vi "AlliGator Export Dataset to TIFF or HDF5.vi"(5 "Dialog?":bool, 6 "Gate Names (Gate)":string[](array[string]), 7 "Destination File Type":string, 8 "error in (no error)":errorcluster, 9 "Channel 2 Image Array":T2[](array[typedef]), 10 "Channel 1 Image Array":T2[](array[typedef]), 11 "Dataset Information":T1={"Single Point Data Path"=path "", "Dataset Timestamp (s)"=0.0, "Current Data"=""}) -> (0 "error out":errorcluster, 1 "Output String":string, 3 "File Path out":path)   [LabVIEW 2021, in "AlliGator Files.lvlib"]
doc: "Saves gate images and dataset information to either a HDF5 file or an image series.\n\n<B>Destination File Type</B>: 'TIFF Series' (Default) or 'HDF5'\n\nNote: TIFF Series does not support dual-gate datasets."
uses:
  AlliGator Files.lvlib
  <vilib>/vision/Image Controls.llb/IMAQ Image.ctl
  AlliGator Current Dataset Information.ctl
  AlliGator Saved TIFF Image Type.ctl
  AlliGator Saved Dataset Information.ctl
  Phasor/Phasor Fluorescence Lifetime Parameters v3.ctl
  Globals, Variables, Constants/AlliGator Variables List.ctl
  <vilib>/Utility/error.llb/Error Cluster From Error Code.vi
  Variant/Variant to Data/Variant to String.vi
  Variant/Variant to Data/Variant to I32.vi
  Globals, Variables, Constants/AlliGator Globals.vi
  <vilib>/ErrorRing/Error Ring.xnode
  GUI/GUI.lvlib
  HDF5/AlliGator HDF5.lvlib
  Strings/Strings.lvlib
  Globals, Variables, Constants/AlliGator Globals, Variables & Constants.lvlib
  Phasor/Phasor.lvlib
  Variant/Variant to Data/Variant to Data.lvlib
panel:
  # "see the AlliGator License on the block diagram (Ctrl+E or Window:Show Block Diagram)"
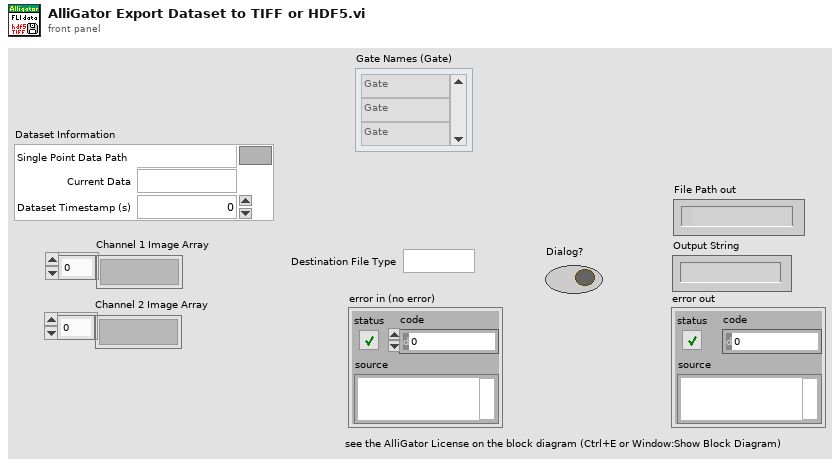
[diagram p1: front panel]
types:
  T1 = typedef "AlliGator Files.lvlib/AlliGator Current Dataset Information.ctl" = cluster{"Single Point Data Path":path, "Dataset Timestamp (s)":dbl, "Current Data":string}
  T2 = typedef "IMAQ Image.ctl" = refnum<image>
  T3 = typedef "Phasor.lvlib/Phasor Fluorescence Lifetime Parameters v3.ctl" = cluster{"# Pixel X":i32, "# Pixel Y":i32, "# Gates":i32, "# Datasets":i32, "Gate Image Exposure":dbl[unit], "Macrotime Gate Separation":dbl[unit], "Nanotime Gate Separation":dbl[unit], "Gate Width":dbl[unit], "Laser Period":dbl[unit], "SYNC Period":dbl[unit], "Gate Image Integration":dbl[unit]}
  T4 = cluster{"Gate Image File Name":string, "File Number Format":string, "Start Index":u32}
  T5 = typedef "AlliGator Files.lvlib/AlliGator Saved TIFF Image Type.ctl" = enum16{"Single Gate", "Sum of All Gates", "Phasor"}
  T6 = typedef "AlliGator Globals, Variables & Constants.lvlib/AlliGator Variables List.ctl" = enum16{"---- GUI ----", "GUI:Initialization Status", "GUI:State Indicators Refnum", "GUI:Original AlliGator Menu Items", "GUI:Current Action Loop State", "GUI:Script in progress", "GUI:Playback", "GUI:Loop Playback", "GUI:Search ROI Used", "GUI:Search ROI", "Decay Graph Max Legend Size", "Intensity Graph Max Legend Size", "Decay Statistics Graph Max Legend Size", "Phasor Graph Max Legend Size", "Phasor Ratio Graph Max Legend Size", "Lifetime Graph Max Legend Size", "---- Files ----", "Files:Export Dataset Frames as Individual Files", "Files:Show Batch Export Help Balloons", "Files:Frames in Dataset", "Files:ptu File Frame Start Indices", "Files:Current Frame in Dataset", "Files:Current Frame Timestamp", "Files:Dataset Loaded", "Files:Dataset Metadata", "Files:Dataset Channel", "Files:Dataset Data Description", "Files:Background Dataset Metadata", "Files:Background Dataset Channel", "Files:Background Dataset Data Description", "Files:Background File Subtraction", "Files:Background File Path", "Files:Background File Pile-up Correction", "Files:Background File Pixel Well Capacity", "Files:Background File Scaling Factor", "Files:Current Dataset Load Settings", "Files:Dataset Path", "Files:ICCD-specific Information", "Files:Macrotime Gate Separation", "------ Python Plugins ------", "Python Plugins:Information", "Python Plugins:Python Session", "Python Plugins:Valid Python Session?", "---- Source Image ----", "Source Image:ROIs", "Source Image:Current ROI", "Source Image:ROI Event Refnum", "X_Source Image:Display Range", "X_Source Image:Palette Information", "X_Source Image:Type of Displayed Image", "X_Time Gate Slider", "Source Image:Palette List", "Source Image:Scale", "Source Image:ROI Overlay Color", "Source Image:Overlay to Erase", "Source Image:Is Displayed Image Accumulated", "Source Image:White Light Image Modified", "Source Image:Mask Image Modified", "---- Image Profile Window ----", "Image Profile:Window Event Refnum", "Image Profile:IntensityType", "Image Profile:Intensity Average Type", "Image Profile:Intensity-weighted SDV", "Image Profile:Box Profile Type", "Image Profile:Window Open", "Image Profile:Plotted Fit Parameter", "------ Phasor Graph -------", "Phasor Graph:Show Line", "---- Phasor Plot ---", "Phasor Plot:Parameters Changed", "Phasor Plot:FLI Dataset Modified since last Calculation", "Phasor Harmonics Data", "Selected Phasor Harmonics", "Phasor Harmonic Manager Event Refnum", "Phasor Plot:ROIs", "Phasor Plot:Current ROI", "Phasor Plot:ROI Event Refnum", "Phasor Plot:Image Reference Points", "Phasor Plot:Computed", "Phasor Plot:Palette Information", "Phasor Plot:Palette List", "Phasor Plot:Phasor Ratio Palette Information", "Phasor Plot:Phasor Ratio Palette List", "Phasor Plot:Image Scale", "Phasor Plot:Image Overlay to Erase", "Phasor Plot:Image Elements to Update", "Phasor Plot:Current Calculation Parameters", "Phasor Plot:Current Calibration Options", "Phasor Plot:Reset Cumulated Phasor Plot", "Phasor Plot:Reference 1", "Phasor Plot:Lifetime Reference 1", "Phasor Plot:Reference 1 Frequency", "Phasor Plot:Reference 2", "Phasor Plot:Lifetime Reference 2", "Phasor Plot:Reference 2 Frequency", "---- Decay Analysis ----", "Number of Selected Decays to Fit", "LS Fit Results", "LAR Fit Results", "BS Fit Results", "Last Decay Max - Min", "Best Fit Parameters", "Best Fit Parameter Names", "Actual Size X", "Actual Size Y", "Binning X", "Binning Y", "Actual # Gates", "Dataset Number", "Gates to...", "Gates Skipped", "Gates to keep", "Gate Step", "Gate Separation", "Reversed Gates", "Pile-up Correction", "Pixel Well Capacity", "Background Subtracted", "Background Subtraction Method", "Background Definition Range", "Background File (deprecated)", "Number of Dataset Accumulated", "Array of Accumulated Dataset Paths", "Do Averaged Datasets", "Destination File Path", "Process Plot Target", "Use 1/D as Phasor Frequency", "---- Decay Fit Parameter Map -----", "Decay Fit Parameter Map:Palette Information", "Decay Fit Parameter Map:Palette List", "---- Parameter Map ----", "Parameter Map:Palette Information", "Parameter Map:Palette List", "------- Local Decay Window ---------", "Local Decay Graph Window:Event Refnum", "Local Decay Graph Window:Use normalized IRF for convolution", "----- Miscellaneous ----", "Misc:Skippable Dialog Windows Status"}
  T7 = typedef "AlliGator Files.lvlib/AlliGator Saved Dataset Information.ctl" = cluster{"Single Dataset Path":path, "Dataset ID in Series (1)":i32, "# Datasets in Series (1)":i32, "Dataset Timestamp (s)":dbl, "Additional Metadata":string, "DAQ Parameters":T3, "Dataset Data Description":string, "X Bin":i32, "Y Bin":i32}
  T8 = typedef "AlliGator Files.lvlib/AlliGator TIFF Series Options.ctl" = cluster{"Gate Image File Name":string, "File Number Format":string, "Start Index":u32, "Save Metadata File":bool, "Compress Image":bool}
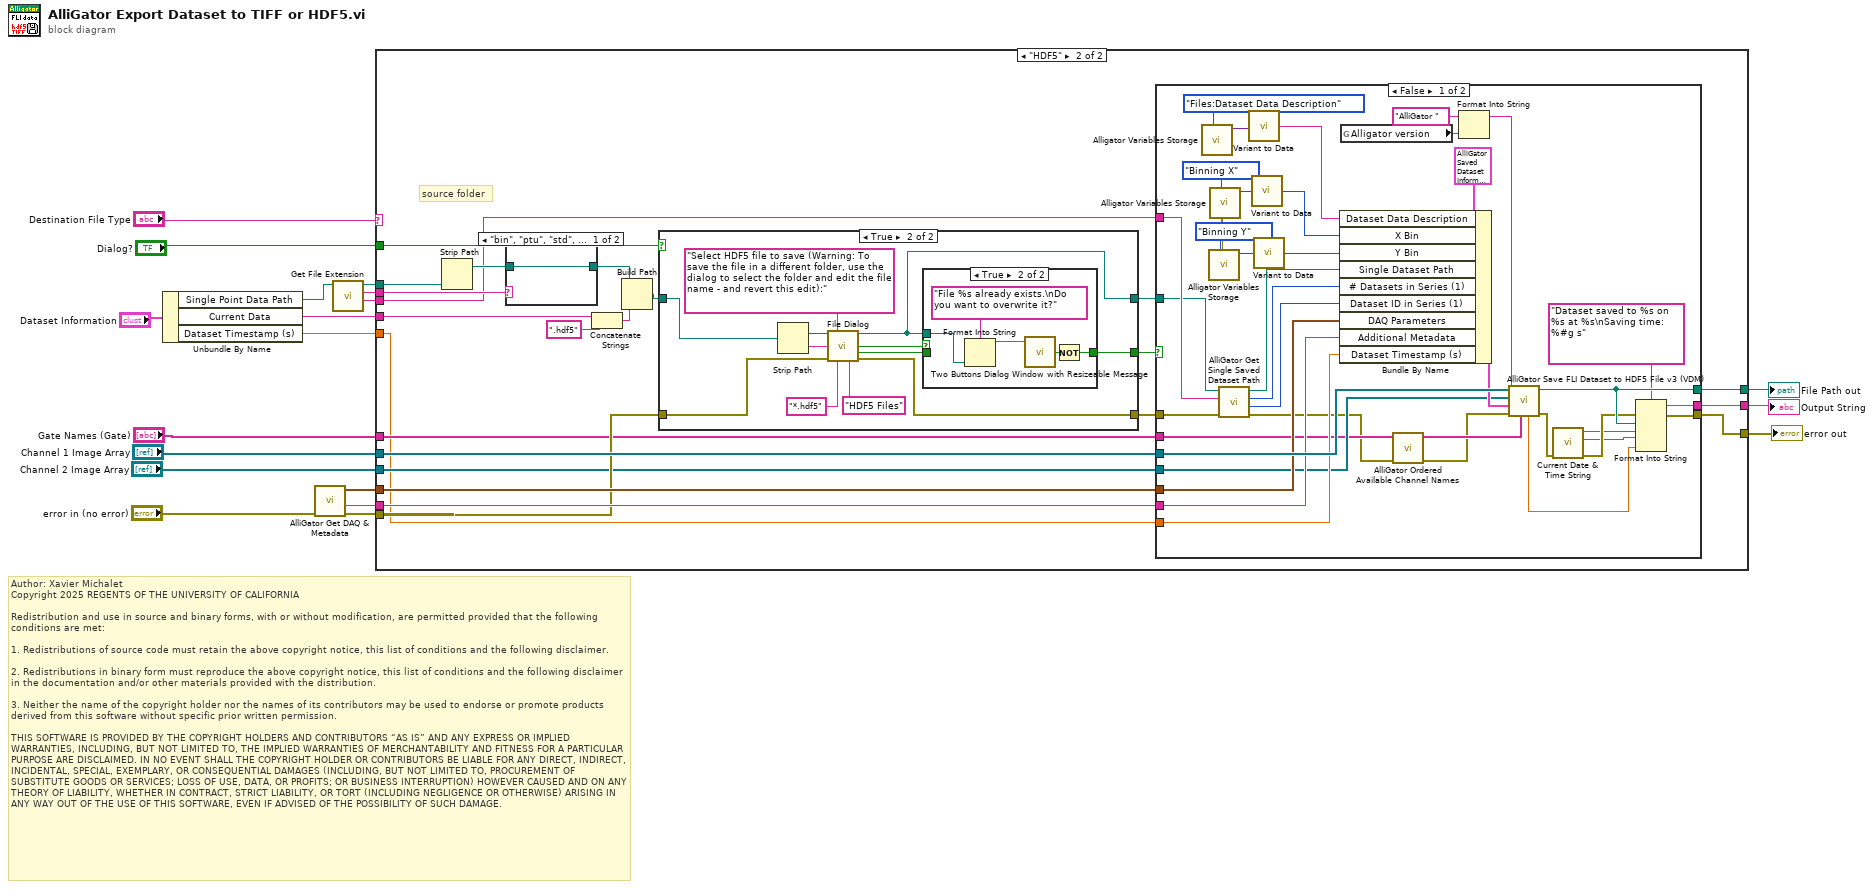
[diagram p0: block diagram]
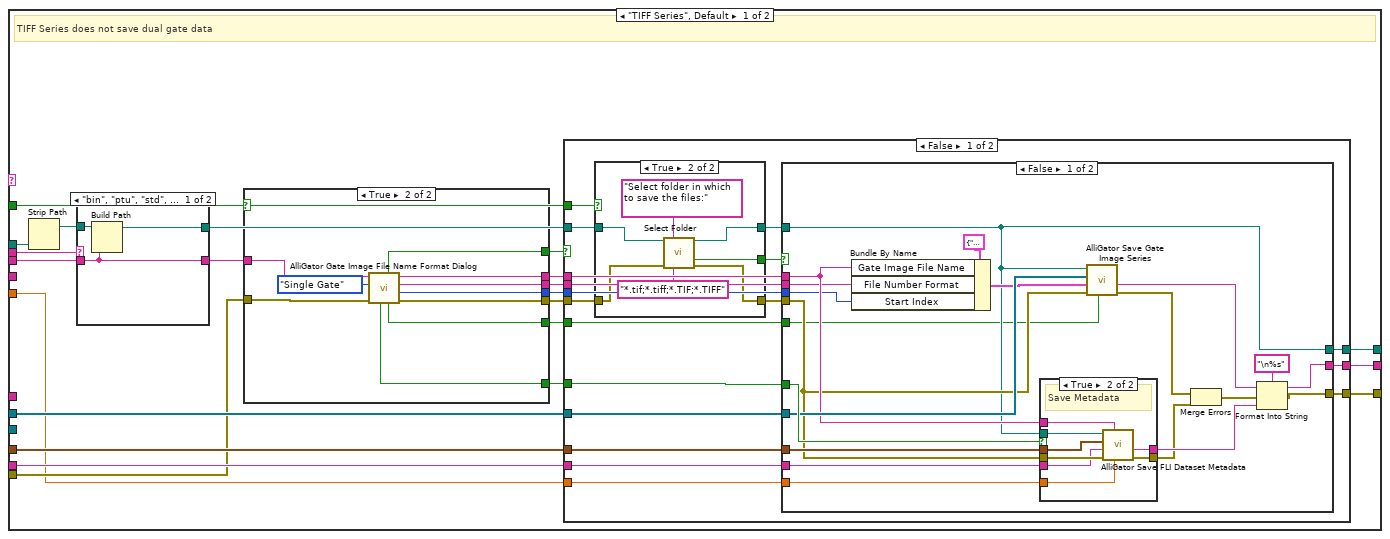
[diagram p2: hidden frame]
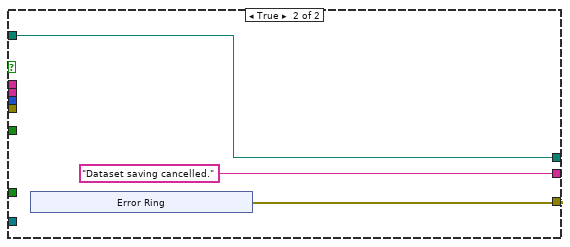
[diagram p4: hidden frame]
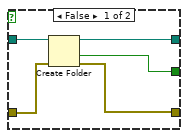
[diagram p5: hidden frame]
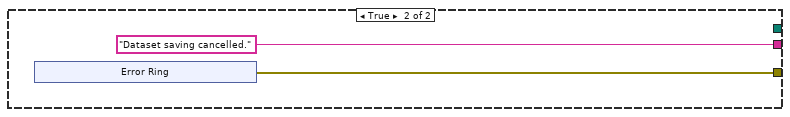
[diagram p6: hidden frame]
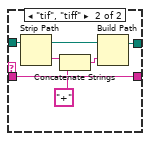
[diagram p7: hidden frame]
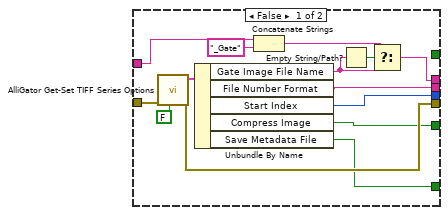
[diagram p8: hidden frame]
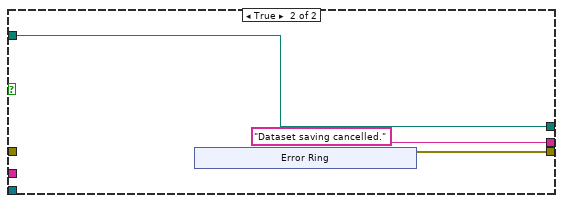
[diagram p9: hidden frame]
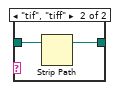
[diagram p12: hidden frame]
diagram:
  # "Author: Xavier Michalet\nCopyright 2025 REGENTS OF THE UNIVERSITY OF CALIFORNIA\n\nRedistribution and use in source and binary forms, with or without modification, are permitted provided that the following conditions are met:\n\n1. Redistributions of source code must retain the above copyright notice, this list of conditions and the following disclaimer.\n\n2. Redistributions in binary form must reproduce the above copyright notice, this list of conditions and the following disclaimer in the documentation and/or other materials provided with the distribution.\n\n3. Neither the name of the copyright holder nor the names of its contributors may be used to endorse or promote products derived from this software without specific prior written permission.\n\nTHIS SOFTWARE IS PROVIDED BY THE COPYRIGHT HOLDERS AND CONTRIBUTORS “AS IS” AND ANY EXPRESS OR IMPLIED WARRANTIES, INCLUDING, BUT NOT LIMITED TO, THE IMPLIED WARRANTIES OF MERCHANTABILITY AND FITNESS FOR A PARTICULAR PURPOSE ARE DISCLAIMED. IN NO EVENT SHALL THE COPYRIGHT HOLDER OR CONTRIBUTORS BE LIABLE FOR ANY DIRECT, INDIRECT, INCIDENTAL, SPECIAL, EXEMPLARY, OR CONSEQUENTIAL DAMAGES (INCLUDING, BUT NOT LIMITED TO, PROCUREMENT OF SUBSTITUTE GOODS OR SERVICES; LOSS OF USE, DATA, OR PROFITS; OR BUSINESS INTERRUPTION) HOWEVER CAUSED AND ON ANY THEORY OF LIABILITY, WHETHER IN CONTRACT, STRICT LIABILITY, OR TORT (INCLUDING NEGLIGENCE OR OTHERWISE) ARISING IN ANY WAY OUT OF THE USE OF THIS SOFTWARE, EVEN IF ADVISED OF THE POSSIBILITY OF SUCH DAMAGE."
  n1 = Unbundle By Name("Dataset Information") -> ("Single Point Data Path"=w3:path, "Current Data"=w2:string, "Dataset Timestamp (s)"=w1:dbl)
  n2 = call "AlliGator Get DAQ & Metadata.vi"("Error In"="error in (no error)") -> ("Error Out"=w13:errorcluster, "Metadata"=w14:string, "DAQ Parameters"=w15:T3)  [unwired: 8 in]
  n3 = call <vilib>:"Get File Extension.vi"("file"=w3) -> ("filename without extension"=w7:string, "lowercase file extension"=w8:string, "dup file"=w9:path)  [unwired: 6 in, 2 out]
  n4 = case shown="\"HDF5\"" "Destination File Type" {
    tunnel: "Channel 1 Image Array" -> [w34 w170]
    tunnel: w15 -> [w33 w169]
    tunnel: w14 -> [w32 w168]
    tunnel: [w37 w167] -> w11
    tunnel: w13 -> [w22 w164]
    tunnel: [w36 w166] -> w18
    tunnel: [w35 w161] -> w12
    tunnel: "Dialog?" -> [w28 w160]
    tunnel: w2 -> [_ w159]
    tunnel: w9 -> [w25 w153]
    tunnel: w8 -> [w26 w155]
    tunnel: w7 -> [w24 w151]
    tunnel: "Channel 2 Image Array" -> [_ w150]
    tunnel: "Gate Names (Gate)" -> [_ w149]
    tunnel: w1 -> [w20 w148]
    frame "TIFF Series", Default {
      # "TIFF Series does not save dual gate data"
      n5 = Strip Path(path=w25) -> (stripped path=w27:path)  [unwired: 1 out]
      n6 = case shown="\"bin\", \"ptu\", \"std\", Default" w26 {
        tunnel: w27 -> [w116 w123]
        tunnel: w24 -> [w115 w122]
        tunnel: [w115 w122] -> w23
        tunnel: [w114 w119] -> w21
        frame "bin", "ptu", "std", Default {
          n7 = Build Path(base path=w116, name or relative path=w115) -> (appended path=w114:path)
        }
        frame "tif", "tiff" {
          n8 = Strip Path(path=w123) -> (stripped path=w121:path, name=w120:string)
          n9 = Concatenate Strings(w120, "+" ("string")) -> (w118:string)
          n10 = Build Path(base path=w121, name or relative path=w118) -> (appended path=w119:path)
        }
      }
      n11 = case shown="True" w28 {
        tunnel: [w133 w147] -> w41
        tunnel: [w132 w146] -> w40
        tunnel: [w130 w145] -> w39
        tunnel: [w131 w144] -> w38
        tunnel: [_ w143] -> w31
        tunnel: [w128 w142] -> w30
        tunnel: [w129 w141] -> w29
        tunnel: w23 -> [w127 w140]
        tunnel: w22 -> [w124 w139]
        frame False {
          n12 = call "AlliGator Get-Set TIFF Series Options.vi"("Set/Get (F)"=FALSE, "error in (no error)"=w124) -> ("error out"=w131:errorcluster, "output cluster out"=w136:T8)  [unwired: 8 in]
          n13 = Unbundle By Name(w136) -> ("Gate Image File Name"=w134:string, "File Number Format"=w132:string, "Start Index"=w130:u32, "Compress Image"=w129:bool, "Save Metadata File"=w128:bool)
          n14 = Concatenate Strings(w127, "_Gate" ("string")) -> (w126:string)
          n15 = Empty String/Path?(string/path=w134) -> (empty?=w135:bool)
          n16 = Select(t=w126, s=w135, f=w134) -> (s? t:f=w133:string)
        }
        frame True {
          n17 = call "AlliGator Gate Image File Name Format Dialog.vi"("error in (no error)"=w139, "Saved TIFF Image"=AlliGator_Saved_TIFF_Image_Type."Single Gate", "Image File Name in"=w140) -> ("error out"=w144:errorcluster, "Start Index out"=w145:u32, "File Number Format out"=w146:string, "Gate Image File Name out"=w147:string, "Compress Image out"=w141:bool, "Cancelled?"=w143:bool, "Save Metadata File out"=w142:bool)  [unwired: 2 in]
        }
      }
      n18 = case shown="False" w31 {
        tunnel: w41 -> [w49 _]
        tunnel: w40 -> [w48 _]
        tunnel: w39 -> [w47 _]
        tunnel: w38 -> [w59 _]
        tunnel: [w58 w109] -> w37
        tunnel: [w56 _] -> w36
        tunnel: [w57 "Dataset saving cancelled."] -> w35
        tunnel: w34 -> [w52 _]
        tunnel: w33 -> [w51 _]
        tunnel: w32 -> [w50 _]
        tunnel: w29 -> [w46 _]
        tunnel: w30 -> [w45 _]
        tunnel: w20 -> [w44 _]
        tunnel: w28 -> [w43 _]
        tunnel: w21 -> [w42 _]
        frame False {
          n19 = case shown="True" w43 {
            tunnel: w59 -> [w99 w107]
            tunnel: [w96 w106] -> w55
            tunnel: [w98 w105] -> w54
            tunnel: [w97 w104] -> w53
            tunnel: w42 -> [w100 w101]
            frame False {
              n20 = Create Folder(path (use dialog)=w100, error in=w99) -> (created path=w96:path, cancelled=w97:bool, error out=w98:errorcluster)  [unwired: 1 in]
            }
            frame True {
              n21 = call "Select Folder"("start path"=w101, "prompt"="Select folder in which to save the files:", "error in"=w107, "pattern (all files)"="*.tif;*.tiff;*.TIF;*.TIFF") -> ("selected path"=w106:path, "cancelled"=w104:bool, "error out"=w105:errorcluster)  [unwired: 8 in, 1 out]
            }
          }
          n22 = case shown="False" w53 {
            tunnel: [w63 w91] -> w58
            tunnel: [w62 "Dataset saving cancelled."] -> w57
            tunnel: [w61 w89] -> w56
            tunnel: w55 -> [w61 w89]
            tunnel: w54 -> [w71 _]
            tunnel: w52 -> [w75 _]
            tunnel: w51 -> [w80 _]
            tunnel: w50 -> [w79 _]
            tunnel: w49 -> [w74 _]
            tunnel: w48 -> [w73 _]
            tunnel: w47 -> [w72 _]
            tunnel: w46 -> [w60 _]
            tunnel: w45 -> [w76 _]
            tunnel: w44 -> [w77 _]
            frame False {
              n23 = Bundle By Name(cluster=T4 {"Gate Image File Name"="", "File Number Format"="", "Start Index"=0} ("File Name Format"), "Gate Image File Name"=w74, "File Number Format"=w73, "Start Index"=w72) -> (w69:T4)
              n24 = case shown="True" w76 {
                tunnel: w80 -> [_ w83]
                tunnel: w79 -> [_ w82]
                tunnel: [_ w88] -> w65
                tunnel: [_ w84] -> w67
                tunnel: w77 -> [_ w81]
                tunnel: w74 -> [_ w87]
                tunnel: w61 -> [_ w86]
                tunnel: w71 -> [_ w85]
                frame False {
                }
                frame True {
                  # "Save Metadata"
                  n25 = call "AlliGator Save FLI Dataset Metadata.vi"("Dataset Timestamp"=w81, "Gate Image File Name"=w87, "error in"=w85, "Metadata"=w82, "DAQ Parameters"=w83, "selected path"=w86) -> ("error out"=w88:errorcluster, "Message"=w84:string)  [unwired: 3 in, 1 out]
                }
              }
              n26 = call "AlliGator Save Gate Image Series.vi"("Compress Image in"=w60, "error in (no error)"=w71, "File Name Format"=w69, "Image Array"=w75, "Folder Path"=w61) -> ("error out"=w78:errorcluster, "Message"=w68:string)  [unwired: 5 in]
              n27 = Merge Errors(w78, w65) -> (w64:errorcluster)
              n28 = Format Into String(format string="\n%s", initial string=w68, error in=w64, w67) -> (resulting string=w62:string, error out=w63:errorcluster)
            }
            frame True {
              n29 = xnode "Error Ring"() -> ("error out"=w91:errorcluster)
            }
          }
        }
        frame True {
          n30 = xnode "Error Ring"() -> ("error out"=w109:errorcluster)
        }
      }
    }
    frame "HDF5" {
      # "source folder"
      n31 = Strip Path(path=w153) -> (stripped path=w152:path)  [unwired: 1 out]
      n32 = case shown="\"bin\", \"ptu\", \"std\", Default" w155 {
        tunnel: [w237 w239] -> w154
        tunnel: w152 -> [w237 w238]
        frame "bin", "ptu", "std", Default {
        }
        frame "tif", "tiff" {
          n33 = Strip Path(path=w238) -> (stripped path=w239:path)  [unwired: 1 out]
        }
      }
      n34 = Concatenate Strings(w159, ".hdf5" ("new ending (none)")) -> (w158:string)
      n35 = Build Path(base path=w154, name or relative path=w158) -> (appended path=w156:path)
      n36 = case shown="True" w160 {
        tunnel: [w218 w227] -> w165
        tunnel: w164 -> [w218 w226]
        tunnel: [w217 w219] -> w163
        tunnel: [_ w224] -> w162
        tunnel: w156 -> [w217 w220]
        frame False {
        }
        frame True {
          n37 = Strip Path(path=w220) -> (stripped path=w222:path, name=w221:string)
          n38 = call "File Dialog"("start path"=w222, "prompt"="Select HDF5 file to save (Warning: To save the file in a different folder, use the dialog to select the folder and edit the file name - and revert this edit):", "default name"=w221, "error in"=w226, "pattern (all files)"="*.hdf5", "pattern label"="HDF5 Files") -> ("selected path"=w219:path, "exists"=w225:bool, "cancelled"=w223:bool, "error out"=w227:errorcluster)  [unwired: 6 in]
          n39 = case shown="True" w225 {
            tunnel: w219 -> [_ w232]
            tunnel: [w231 w235] -> w224
            tunnel: w223 -> [w231 _]
            frame False {
            }
            frame True {
              n40 = Format Into String(format string="File %s already exists.\nDo you want to overwrite it?", w232) -> (resulting string=w234:string)  [unwired: 2 in, 1 out]
              n41 = call "Two Buttons Dialog Window with Resizeable Message.vi"("Message"=w234) -> ("OK?"=w236:bool)  [unwired: 8 in]
              n42 = Not(x=w236) -> (.not. x?=w235:bool)
            }
          }
        }
      }
      n43 = case shown="False" w162 {
        tunnel: w170 -> [w209 _]
        tunnel: w169 -> [w192 _]
        tunnel: w168 -> [w191 _]
        tunnel: [w207 w211] -> w167
        tunnel: [w208 w212] -> w166
        tunnel: w165 -> [w204 _]
        tunnel: w163 -> [w201 w212]
        tunnel: [w205 "Dataset saving cancelled."] -> w161
        tunnel: w151 -> [w203 _]
        tunnel: w148 -> [w190 _]
        tunnel: w150 -> [w188 _]
        tunnel: w149 -> [w175 _]
        frame False {
          n44 = call "Alligator Variables Storage.vi"("AlliGator Variable"=AlliGator_Variables_List."Files:Dataset Data Description" ("Alligator Variable")) -> ("Data out"=w186:variant)  [unwired: 8 in, 2 out]
          n45 = call "Alligator Variables Storage.vi"("AlliGator Variable"=AlliGator_Variables_List."Binning X" ("Alligator Variable")) -> ("Error Out"=w182:errorcluster, "Data out"=w181:variant)  [unwired: 8 in, 1 out]
          n46 = call "Alligator Variables Storage.vi"("AlliGator Variable"=AlliGator_Variables_List."Binning Y" ("Alligator Variable"), "Error In"=w182) -> ("Data out"=w180:variant)  [unwired: 7 in, 2 out]
          n47 = call "AlliGator Get Single Saved Dataset Path.vi"("error in (no error)"=w204, "Original Dataset Name without Extension"=w203, "Single Dataset Path"=w201) -> ("error out"=w173:errorcluster, "Current Frame in Dataset"=w193:i32, "# Frames in Dataset"=w194:i32, "Single Dataset Path"=w187:path)  [unwired: 5 in]
          n48 = call-poly "Variant to Data.vi"("Variant"=w186) -> ("String"=w179:string)  [unwired: 8 in]
          n49 = call-poly "Variant to Data.vi"("Variant"=w181) -> ("Value"=w178:i32)  [unwired: 8 in]
          n50 = call-poly "Variant to Data.vi"("Variant"=w180) -> ("Value"=w177:i32)  [unwired: 8 in]
          n51 = Bundle By Name(cluster=T7 {"Single Dataset Path"=path "", "Dataset ID in Series (1)"=1, "# Datasets in Series (1)"=1, "Dataset Timestamp (s)"=0.0, "Additional Metadata"="", "DAQ Parameters"={"# Pixel X"=0, "# Pixel Y"=0, "# Gates"=0, "# Datasets"=0, "Gate Image Exposure"=0.0, "Macrotime Gate Separation"=0.0, "Nanotime Gate Separation"=0.0, "Gate Width"=0.0, "Laser Period"=0.0, "SYNC Period"=0.0, "Gate Image Integration"=0.0}, "Dataset Data Description"="", "X Bin"=0, "Y Bin"=0} ("Dataset Information"), "Dataset Data Description"=w179, "X Bin"=w178, "Y Bin"=w177, "Single Dataset Path"=w187, "# Datasets in Series (1)"=w194, "Dataset ID in Series (1)"=w193, "DAQ Parameters"=w192, "Additional Metadata"=w191, "Dataset Timestamp (s)"=w190) -> (w195:T7)
          n52 = global read "AlliGator Globals.vi" "Alligator version"() -> (w189:string)
          n53 = call "AlliGator Ordered Available Channel Names.vi"("error in (no error)"=w173, "Channel Names"=w175) -> ("error out"=w172:errorcluster, "Ordered Channel Names"=w174:string[])  [unwired: 8 in]
          n54 = Format Into String(initial string="AlliGator ", w189) -> (resulting string=w176:string)  [unwired: 2 in, 1 out]
          n55 = call "AlliGator Save FLI Dataset to HDF5 File v3 (VDM).vi"("Gate Names (Gate)"=w174, "Software + Version"=w176, "Error In"=w172, "Dataset Information"=w195, "Channel 2 Gate Image Array"=w188, "Channel 1 Gate Image Array"=w209) -> ("Error Out"=w200:errorcluster, "File Path out"=w208:path, "Time (s)"=w171:dbl)  [unwired: 3 in]
          n56 = call "Current Date & Time String.vi"("Error In"=w200) -> ("Error Out"=w199:errorcluster, "time string"=w197:string, "date string"=w198:string)  [unwired: 8 in]
          n57 = Format Into String(format string="Dataset saved to %s on %s at %s\nSaving time: %#g s", error in=w199, w208, w198, w197, w171) -> (resulting string=w205:string, error out=w207:errorcluster)  [unwired: 1 in]
        }
        frame True {
          n58 = xnode "Error Ring"() -> ("error out"=w211:errorcluster)
        }
      }
    }
  }
  "error out" <- w11
  "Output String" <- w12
  "File Path out" <- w18
